vi "E1_Suma.vi"() -> ()   [LabVIEW 2020]
panel:
  out "Y":dbl
  in  "B":dbl
  in  "A":dbl
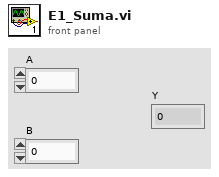
[diagram p1: front panel]
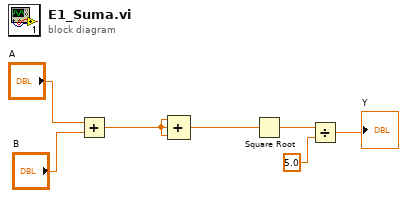
[diagram p0: block diagram]
diagram:
  n1 = Add(x="A", y="B") -> (x+y=w2:dbl)
  n2 = Compound Arithmetic op=ADD(w2, w2, w2) -> (w1:dbl)
  n3 = Square Root(x=w1) -> (sqrt(x)=w5:dbl)
  n4 = Divide(x=w5, y=5.0) -> (x/y=→"Y":dbl)
